vi "Run_Sequence.vi"(0 "Input Sequence":cluster{string, string[], dbl[], dbl}[](array[cluster]), 1 "Alias Table":string[][](array[string]), 2 "API Function Array":cluster{string, "VI Reference":refnum<vi>}[](array[cluster]), 3 "Debug":bool=TRUE, 4 "Resume":bool) -> ()   [LabVIEW 2011]
doc: "This is the highest level VI designed for running growth sequences. It will display all currently running commands, allowing the user to switch between them to view their various statuses. Additionally, if the current command calls for user input before continuing, this VI will display a \"Continue?\" button and enable the \"Waiting for Input...\" indicator. \"Abort Sequence\" will terminate the sequence regardless of the current position and reinitialize the MOCVD system, while \"Pause Sequence\" will end the sequence while leaving the current external hardware state intact. This allows the user to return to the editor, make any applicable changes, and resume the sequence where it was left off."
uses:
  <vilib>/Platform/TimedLoop/XDataNode/nitl_modes.ctl
  <vilib>/Platform/TimedLoop/XDataNode/timing_clust.ctl
  <vilib>/Platform/TimedLoop/XDataNode/wakeup.ctl
  low_level_proc/globals.vi
  Flow_Globals.vi
  <vilib>/Platform/TimedLoop/XDataNode/XDataNode.xnode
  <vilib>/Platform/TimedLoop/XDataNode/XDNodeRunTimeDep.lvlib
panel:
  out "Prev":string
  out "Ended Loop":cluster{string, "Position":i32}[](array[cluster])
  in  "Log/Flow Tabs":T1(tab)=enum."Flow Targets"
  out "Log":string
  out "As":dbl caption="As (0-10 sscm)"
  out "P":dbl caption="P (0-100 sscm)"
  out "In":dbl caption="In (0-10 sscm)"
  out "Ga 3":dbl caption="Ga 3 (0-1000 sscm)"
  out "Ga 2":dbl caption="Ga 2 (0-10 sscm)"
  out "Ga 1":dbl caption="Ga 1 (0-10 sscm)"
  out "Al":dbl caption="Al (0-100 sscm)"
  out "N2":dbl caption="N2 (0-10 slm)"
  out "H2":dbl caption="H2 (0-10 slm)"
  in  "H2/N2 View":bool
  out "As A":dbl caption="As (0-10 sscm)"
  out "P A":dbl caption="P (0-100 sscm)"
  out "In A":dbl caption="In (0-10 sscm)"
  out "Ga 3 A":dbl caption="Ga 3 (0-1000 sscm)"
  out "Ga 2 A":dbl caption="Ga 2 (0-10 sscm)"
  out "Ga 1 A":dbl caption="Ga 1 (0-10 sscm)"
  out "Al A":dbl caption="Al (0-100 sscm)"
  out "N2 A":dbl caption="N2 (0-10000 sscm)"
  out "H2 A":dbl caption="H2 (0-10000 sscm)"
  in  "Heater":bool
  in  "Spinner":bool
  in  "HS Remote":bool caption="Remote"
  out "Position":i32
  out "Ping Time":dbl
  out "Waiting for Input...":bool
  in  "Display Tabs":enum32{"Default", "Time", "Temperature", "Loop"}(tab)
  out "Total Time":u8(slide) caption="Total Time:" scale=0.0..100.0
  out "CE Time":u8(slide) caption="Event Time:" scale=0.0..100.0
  out "Total Time Remaining String":string="00:00" caption="Remaining:"
  out "CE Time Remaining String":string="00:00" caption="Remaining:"
  out "Current Event:":string
  out "Current Temperature (C)":dbl
  out "Target (C)":dbl
  out "Temperature":u8(slide) caption="Temperature:" scale=0.0..100.0
  out "Iteration":string
  in  "Status Tabs":enum32{"Default", "Status", "Prompt"}(tab)
  out "Comment:":string
  out "Selected Event:":string
  in  "Go To Next Step":bool
  out "Prompt:":string
  in  "Continue":bool
  in  "Active Events":i32(listbox)=-1
  in  "Abort":bool
  in  "Pause":bool
  out "Error Out":errorcluster caption="error out"
  out "Running":bool caption="Sequence in Progress..."
  # "Loop Iteration:"
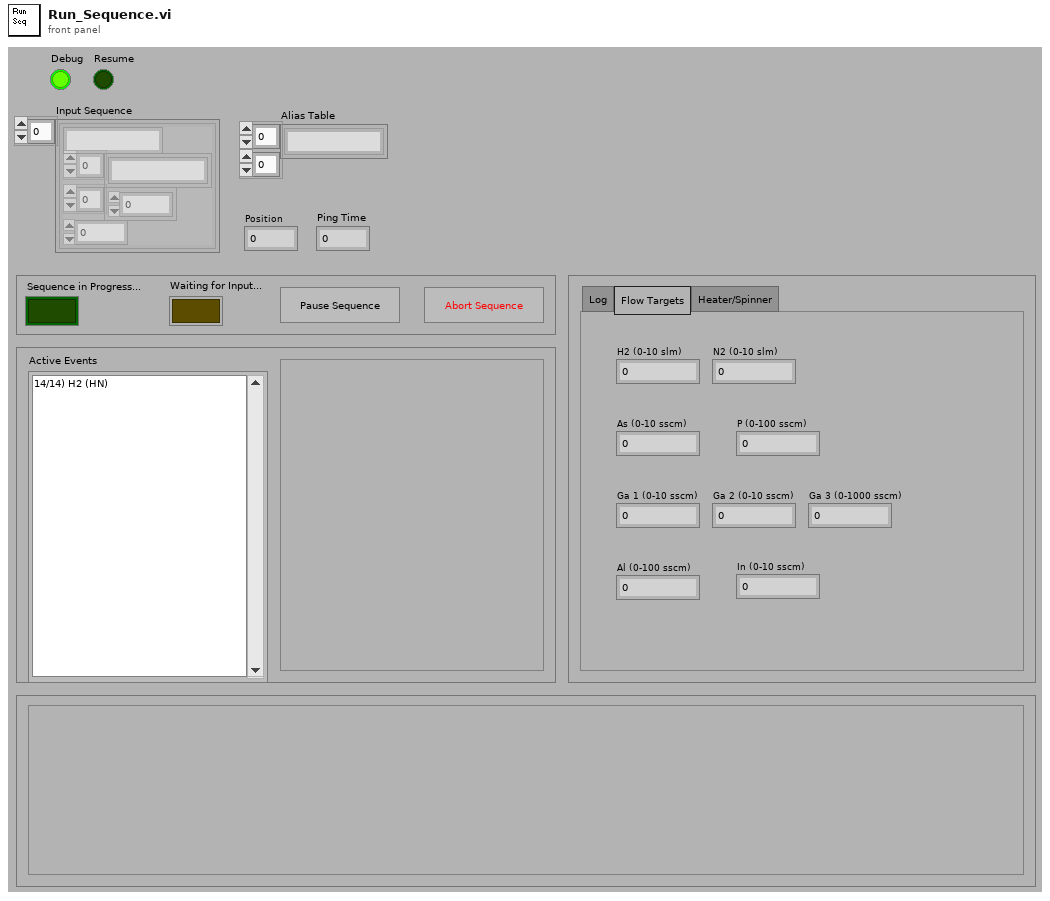
[diagram p1: front panel]
types:
  T1 = enum32{"Log", "Flow Targets", "Detected Flows", "Heater/Spinner"}
  T2 = typedef "XDNodeRunTimeDep.lvlib/nitl_modes.ctl" = enum32{"No Change", "Process missed periods, maintain original phase", "Discard missed periods, maintain original phase", "Process missed periods, ignore original phase", "Discard missed periods, ignore original phase"}
  T3 = enum8{"Enabled", "Disabled", "Disabled and Grayed Out"}
  T4 = typedef "XDNodeRunTimeDep.lvlib/timing_clust.ctl" = cluster{"Expected End [f-1]":u64, "Actual End [f-1]":u64, "Finished Late? [f-1]":bool, "Expected End [i-1]":u64, "Actual End [i-1]":u64, "Finished Late? [i-1]":bool, "Expected Start [i]":u64, "Actual Start [i]":u64, "Expected Start [f]":u64, "Actual Start [f]":u64, "Source Name":string, "Structure Name":string, "Period":i64, "Deadline":i64, "Offset":i64, "Start":i64, "Priority":i32, "Timeout":i32, "Mode":T2, "Wakeup Reason":T5, "Error":errorcluster, "Source Type":string, "Secondary Source Type":string, "Global End Time":u64, "Global Start Time":u64, "Frame Duration":u64, "Iteration Duration":u64, "Assigned CPU":i32, "I/O Scan Engine Mode":u32}
  T5 = typedef "XDNodeRunTimeDep.lvlib/wakeup.ctl" = enum32{"Normal", "Aborted", "Asynchronous wakeup", "Timing source error", "Timed loop error", "Timeout"}
  T6 = enum16{"Normal", "Blocking", "Wait for Input", "Loop"}
  T7 = cluster{"Argument List Out":string[], "Status Out":string}[]
  T8 = cluster{"Total Time Remaining":dbl, "Total Time":dbl, "Current Time Remaining":dbl, "Current Event Time":dbl}
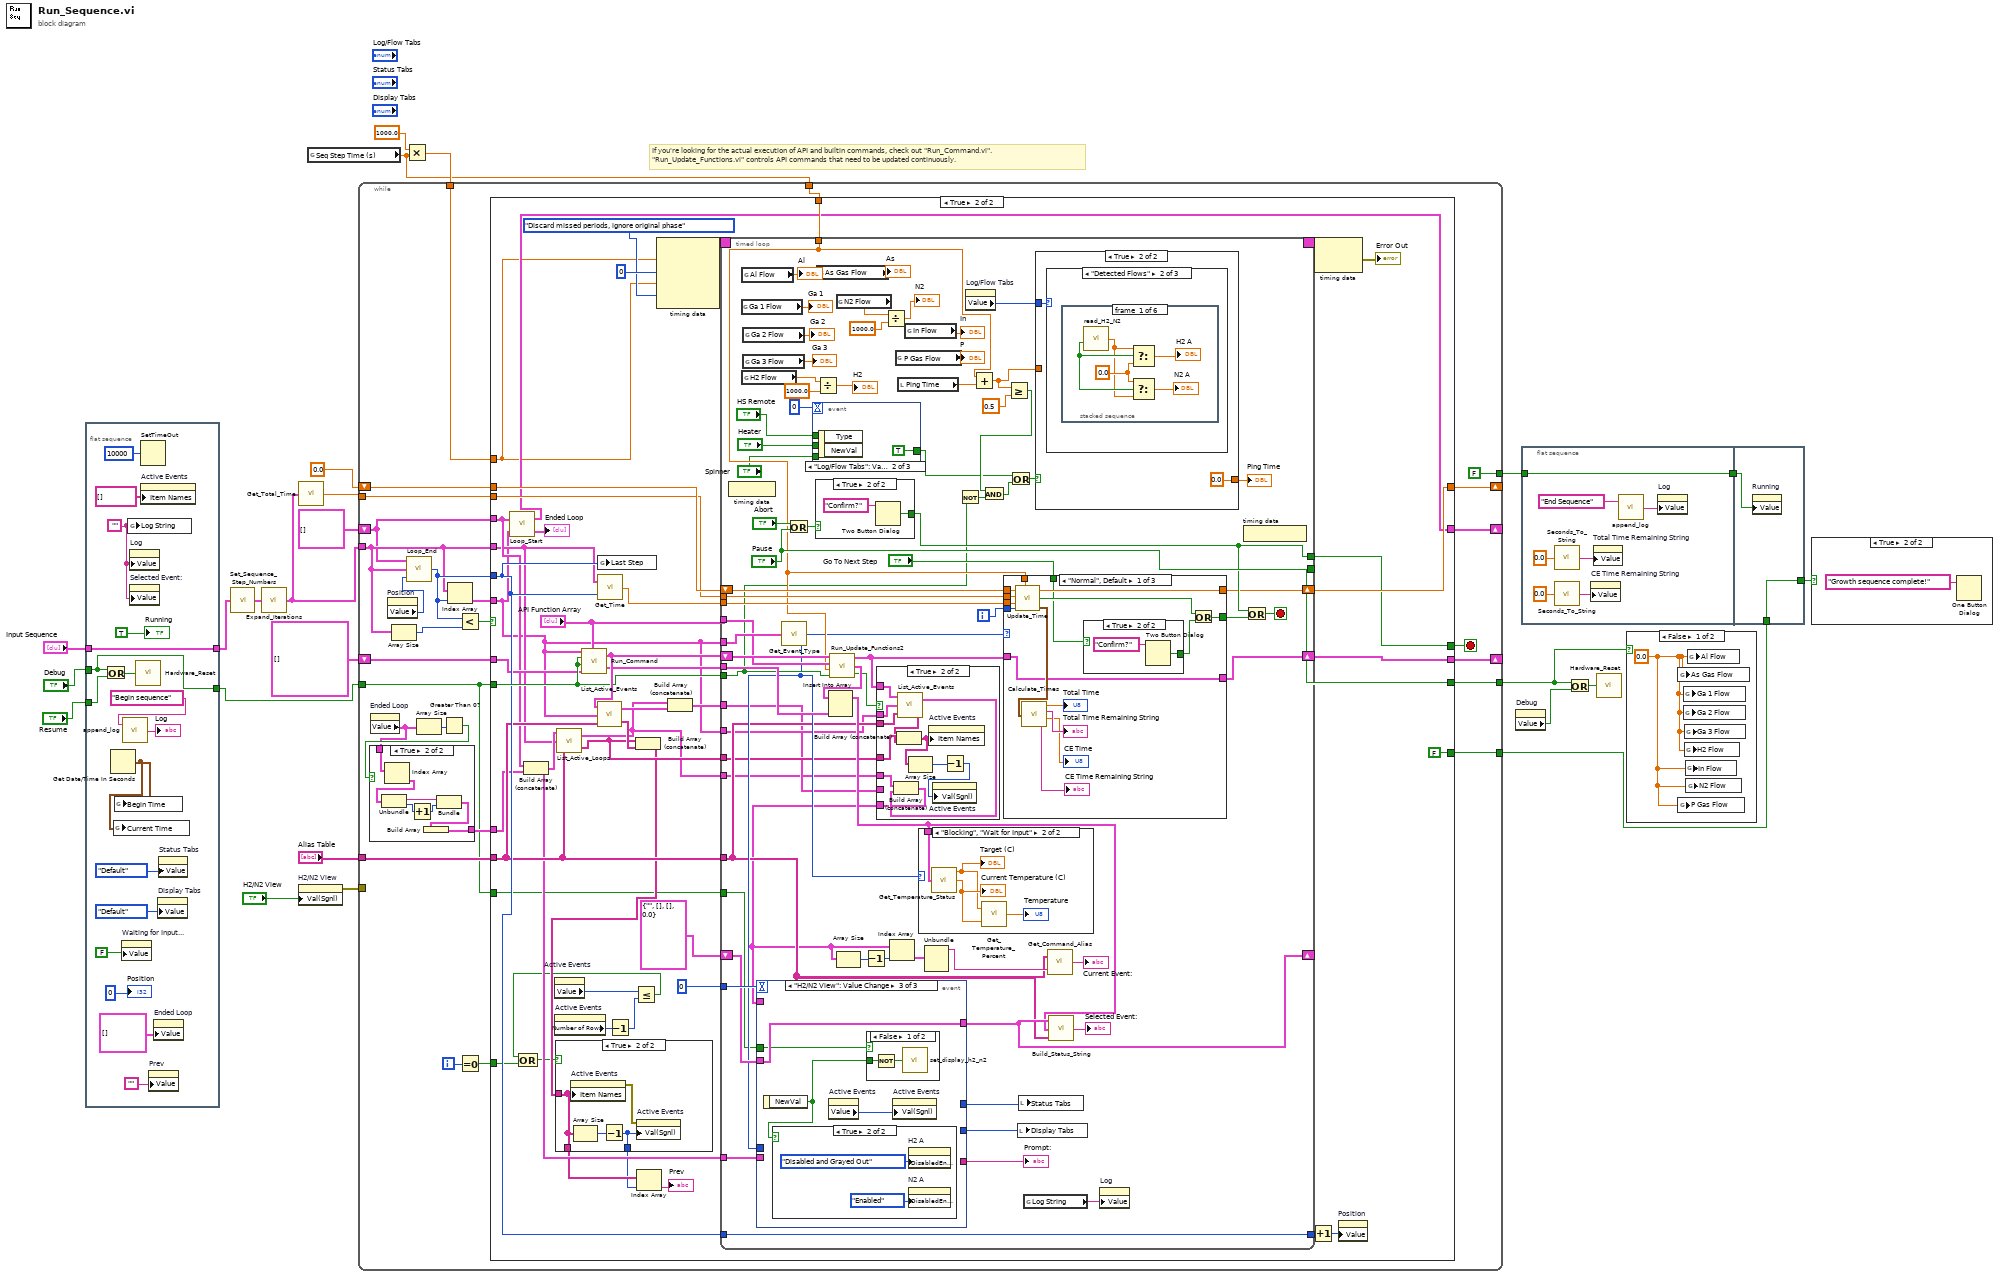
[diagram p0: block diagram]
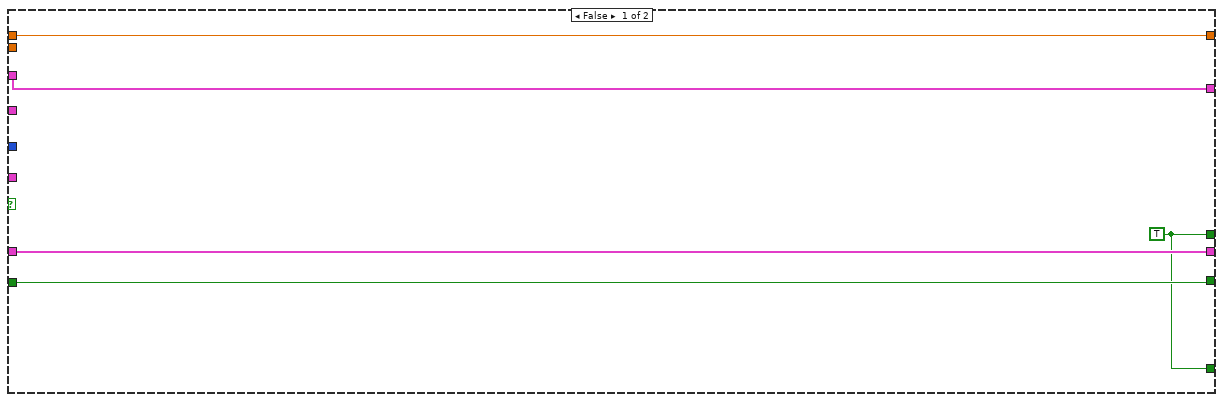
[diagram p4: hidden frame]
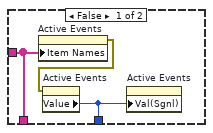
[diagram p5: hidden frame]
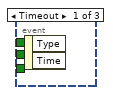
[diagram p7: hidden frame]
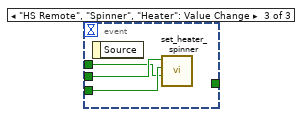
[diagram p8: hidden frame]
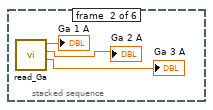
[diagram p12: hidden frame]
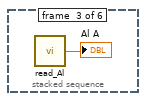
[diagram p13: hidden frame]
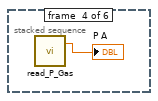
[diagram p14: hidden frame]
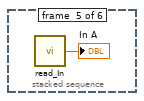
[diagram p15: hidden frame]
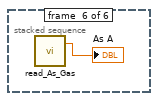
[diagram p16: hidden frame]
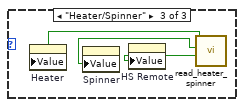
[diagram p17: hidden frame]
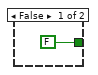
[diagram p18: hidden frame]
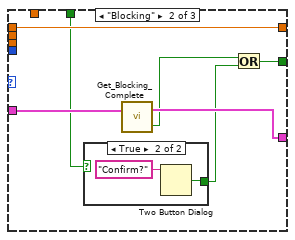
[diagram p19: hidden frame]
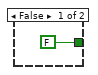
[diagram p20: hidden frame]
diagram:
  # "If you're looking for the actual execution of API and builtin commands, check out \"Run_Command.vi\".\n\"Run_Update_Functions.vi\" controls API commands that need to be updated continuously."
  n1 = flat-sequence {
    tunnel: [w41] -> w3
    tunnel: "Input Sequence" -> [w41]
    tunnel: "Debug" -> [w29]
    tunnel: [w29] -> w19
    tunnel: "Resume" -> [w31]
    frame #0 {
      w36 = ""
      n2 = Or(x=w29, y=w31) -> (x .or. y?=w30:bool)
      n3 = Get Date/Time In Seconds() -> (seconds since 1Jan1904=w37:timestamp)
      n4 = global write "globals.vi" "Current Time"(w37) -> ()
      n5 = global write "globals.vi" "Begin Time"(w37) -> ()
      n6 = property on="Waiting for Input..." class="Bool (strict)"("Value"=FALSE ("Waiting for Input...")) -> ()  [unwired: 2 in, 2 out]
      n7 = call "append_log.vi"("New Log String"="Begin sequence") -> ("Log"=→"Log":string)  [unwired: 1 in]
      n8 = global write "globals.vi" "Log String"(w36) -> ()
      n9 = property on="Log" class="Str"("Value"=w36) -> ()  [unwired: 2 in, 2 out]
      n10 = property on="Selected Event:" class="Str"("Value"=w36) -> ()  [unwired: 2 in, 2 out]
      n11 = call "Hardware_Reset.vi"("Debug"=w30) -> ()  [unwired: 1 out]
      n12 = SetTimeOut(1:10000 ("new timeout (10000)")) -> ()  [unwired: 1 out]
      n13 = property on="Active Events" class="LstBox (strict)"("Item Names"=string[] []) -> ()  [unwired: 2 in, 2 out]
      n14 = property on="Prev" class="Str"("Value"="") -> ()  [unwired: 2 in, 2 out]
      n15 = property on="Ended Loop" class="Arr (strict)"("Value"=cluster{string, "Position":i32}[] [] ("Ended Loop")) -> ()  [unwired: 2 in, 2 out]
      n16 = property on="Display Tabs" class="TabCtl (strict)"("Value"=enum32{"Default", "Time", "Temperature"}."Default" ("Display Tabs")) -> ()  [unwired: 2 in, 2 out]
      n17 = property on="Status Tabs" class="TabCtl (strict)"("Value"=enum32{"Default", "Status", "Prompt"}."Default" ("Status Tabs")) -> ()  [unwired: 2 in, 2 out]
      "Running" <- TRUE ("Sequence in Progress...")
      "Position" <- 0 ("Position")
    }
  }
  n18 = call "Set_Sequence_Step_Numbers.vi"("Input Sequence"=w3) -> ("Output Sequence"=w4:cluster{string, string[], dbl[], dbl}[])
  n19 = call "Expand_Iterations.vi"("Input Sequence"=w4) -> ("Output Sequence"=w9:cluster{string, string[], dbl[], dbl}[])
  n20 = property on="H2/N2 View" class="Bool (strict)"("Val(Sgnl)"="H2/N2 View") -> (error out=w2:errorcluster)  [unwired: 2 in, 1 out]
  n21 = call "Get_Total_Time.vi"("Input Sequence"=w9) -> ("Total Time"=w24:dbl)
  n22 = global read "globals.vi" "Seq Step Time (s)"() -> (w12:dbl)
  n23 = Multiply(x=1000.0, y=w12) -> (x*y=w14:dbl)
  n24 = while {
    tunnel: w24 -> [w66]
    tunnel: [FALSE ("Sequence in Progress...")] -> w20
    tunnel: w9 -> [w53]
    shift-right: [w67] -> _
    shift-left: 0.0 -> [w68]
    tunnel: [w65] -> w5
    shift-right: [w64] -> _
    shift-left: cluster{string, string[], dbl[], dbl}[] [] ("Update Functions Out") -> [w62]
    tunnel: w19 -> [w42]
    tunnel: w14 -> [w63]
    tunnel: "Alias Table" -> [w61]
    tunnel: w12 -> [w60]
    shift-right: [w58] -> _
    shift-left: cluster{string, "Position":i32}[] [] ("appended array") -> [w51]
    tunnel: [w50] -> w8
    tunnel: w2 -> [_]
    i -> [w44]
    stop <- w49 stop-if-true
    n25 = property on="Ended Loop" class="Arr (strict)"() -> ("Value"=w46:cluster{string, "Position":i32}[])  [unwired: 2 in, 2 out]
    n26 = property on="Position" class="DigNum (strict)"() -> ("Value"=w59:i32)  [unwired: 2 in, 2 out]
    n27 = Array Size(array=w53) -> (size(s)=w52:i32)
    n28 = call "Loop_End.vi"("Position In"=w59, "Input Sequence"=w53, "Loop Count In"=w51) -> ("Position Out"=w54:i32)
    n29 = Array Size(array=w46) -> (size(s)=w48:i32)
    n30 = Greater Than 0?(x=w48) -> (x > 0?=w47:bool)
    n31 = case shown="True" w47 {
      tunnel: w46 -> [w69 w76]
      tunnel: [w69 w70] -> w45
      frame False {
      }
      frame True {
        n32 = Index Array(array=w76) -> (element=w75:cluster{string, "Position":i32})  [unwired: 1 in]
        n33 = Unbundle(w75) -> (w72:string, "Position"=w74:i32)
        n34 = Increment(x=w74) -> (x+1=w73:i32)
        n35 = Bundle(w72, w73) -> (w71:cluster{string, i32})  [unwired: 1 in]
        n36 = Build Array(w71) -> (w70:cluster{string, i32}[])
      }
    }
    n37 = Index Array(array=w53, index=w54) -> (element=w56:cluster{string, string[], dbl[], dbl})
    n38 = Less?(x=w54, y=w52) -> (x < y?=w55:bool)
    n39 = Equal To 0?(x=w44) -> (x = 0?=w43:bool)
    n40 = case shown="True" w55 {
      tunnel: w68 -> [w78 w128]
      tunnel: [w78 w127] -> w67
      tunnel: w66 -> [_ w126]
      tunnel: [w79 w125] -> w65
      tunnel: [w81 w124] -> w64
      tunnel: w63 -> [_ w106]
      tunnel: w62 -> [w81 w105]
      tunnel: w61 -> [_ w104]
      tunnel: w60 -> [_ w117]
      tunnel: w42 -> [w79 w115]
      tunnel: w53 -> [_ w97]
      tunnel: w54 -> [_ w111]
      tunnel: w51 -> [w80 w103]
      tunnel: [w80 w108] -> w58
      tunnel: [w77 w112] -> w49
      tunnel: w56 -> [_ w92]
      tunnel: [w77 FALSE ("T button?")] -> w50
      tunnel: w45 -> [_ w102]
      tunnel: w43 -> [_ w94]
      tunnel: w42 -> [_ w82]
      frame False {
        w77 = TRUE ("T button?")
      }
      frame True {
        n41 = call "Loop_Start.vi"("Command"=w92, "Loop Count In"=w103) -> ("Ended Loop"=→"Ended Loop":cluster{string, "Position":i32}[], "Loop Count Out"=w108:cluster{string, "Position":i32}[])
        n42 = Build Array (concatenate)(w103, w102) -> (w98:cluster{string, "Position":i32}[])
        n43 = property on="Active Events" class="LstBox (strict)"() -> ("Value"=w85:i32)  [unwired: 2 in, 2 out]
        n44 = property on="Active Events" class="LstBox (strict)"() -> ("Number of Rows"=w95:u32)  [unwired: 2 in, 2 out]
        n45 = call "List_Active_Loops.vi"("Alias Table"=w104, "Input Sequence"=w97, "Loop Count In"=w98) -> ("Item List"=w93:string[], "Loops Out"=w87:cluster{string, string[], dbl[], dbl}[])
        n46 = call "Run_Command.vi"("Event"=w92, "Debug Mode"=w115, "Realtime Debug"=w115, "Update Functions In"=w105, "API Function Array"="API Function Array") -> ("Update Functions Out"=w118:cluster{string, string[], dbl[], dbl}[], "Status Array"=w114:cluster{string[], "Status Out":string}[])
        n47 = call "List_Active_Events.vi"("Alias Table"=w104, "Current Event"=w92, "Update Functions In"=w118) -> ("Item List"=w101:string[], "Update Functions Out"=w100:cluster{string, string[], dbl[], dbl}[])
        n48 = global write "globals.vi" "Last Step"(w111) -> ()
        n49 = call "Get_Time.vi"("Index"=w111, "Input Sequence"=w97) -> ("Time (s)"=w123:dbl)
        n50 = Decrement(x=w95) -> (x-1=w84:u32)
        n51 = Less Or Equal?(x=w85, y=w84) -> (x <= y?=w83:bool)
        n52 = Compound Arithmetic op=OR(w83, w94) -> (w86:bool)
        n53 = Build Array (concatenate)(w93, w101) -> (w91:string[])
        n54 = case shown="True" w86 {
          tunnel: w91 -> [w132 w135]
          tunnel: [w132 w135] -> w89
          tunnel: [w131 w134] -> w88
          frame False {
            n55 = property on="Active Events" class="LstBox (strict)"("Item Names"=w132) -> (error out=w133:errorcluster)  [unwired: 2 in, 1 out]
            n56 = property on="Active Events" class="LstBox (strict)"(error in=w133) -> ("Value"=w131:i32)  [unwired: 1 in, 2 out]
            n57 = property on="Active Events" class="LstBox (strict)"("Val(Sgnl)"=w131) -> ()  [unwired: 2 in, 2 out]
          }
          frame True {
            n58 = property on="Active Events" class="LstBox (strict)"("Item Names"=w135) -> (error out=w136:errorcluster)  [unwired: 2 in, 1 out]
            n59 = Array Size(array=w135) -> (size(s)=w137:i32)
            n60 = Decrement(x=w137) -> (x-1=w134:i32)
            n61 = property on="Active Events" class="LstBox (strict)"(error in=w136, "Val(Sgnl)"=w134) -> ()  [unwired: 1 in, 2 out]
          }
        }
        n62 = Index Array(array=w89, index=w88) -> (element=→"Prev":string)
        n63 = node-c288(w106, i64 0 ("Offset"), w106, nitl_modes."Discard missed periods, ignore original phase" ("Mode")) -> (w130:T4)
        n64 = Build Array (concatenate)(w87, w100) -> (w99:cluster{string, string[], dbl[], dbl}[])
        n65 = timed-loop {
          timing: w130 -> [_]
          timing-out: [_] -> w129
          tunnel: w123 -> [w197]
          tunnel: w126 -> [w198]
          shift-right: [w196] -> w127
          shift-left: w128 -> [w199]
          tunnel: [w207] -> w112
          tunnel: ["Pause"] -> w125
          shift-right: [w191] -> w124
          shift-left: w118 -> [w192]
          tunnel: w115 -> [w178]
          tunnel: 0 -> [w206]
          tunnel: w104 -> [w153]
          shift-right: [w185] -> _
          shift-left: cluster{string, string[], dbl[], dbl} {"", [], [], 0.0} -> [w202]
          tunnel: w92 -> [w201]
          tunnel: w99 -> [w150]
          tunnel: "API Function Array" -> [w190]
          tunnel: w117 -> [w180]
          tunnel: w114 -> [w183]
          tunnel: w111 -> [w174]
          tunnel: [w174] -> w113
          tunnel: w98 -> [w156]
          tunnel: w93 -> [w152]
          tunnel: w92 -> [w151]
          tunnel: w87 -> [w148]
          tunnel: w82 -> [w141]
          i -> [w181]
          stop <- w208 stop-if-true
          n66 = node-c288() -> ()  [unwired: 1 out]
          n67 = global read "Flow_Globals.vi" "Ga 1 Flow"() -> (→"Ga 1":dbl)
          n68 = global read "Flow_Globals.vi" "Al Flow"() -> (→"Al":dbl)
          n69 = global read "Flow_Globals.vi" "H2 Flow"() -> (w147:dbl)
          n70 = global read "Flow_Globals.vi" "Ga 2 Flow"() -> (→"Ga 2":dbl)
          n71 = global read "Flow_Globals.vi" "Ga 3 Flow"() -> (→"Ga 3":dbl)
          n72 = call "Get_Event_Type.vi"("Event"=w201) -> ("Event Type"=w177:T6)
          n73 = Or(x="Abort", y="Pause") -> (x .or. y?=w189:bool)
          n74 = event shown="[1] \"Log/Flow Tabs\": Value Change" {
            selector: _ -> [_ _ _]
            dyn-events: _ -> [_ _ _]
            timeout: 0 -> [_ _ _]
            tunnel: [_ TRUE _] -> w161
            tunnel: "HS Remote" -> [_ _ w224]
            tunnel: "Spinner" -> [_ _ w226]
            tunnel: "Heater" -> [_ _ w225]
            event Timeout {
              n75 = event-data() -> ()  [unwired: 1 in, 2 out]
            }
            event "Log/Flow Tabs": Value Change {
              n76 = event-data() -> ()  [unwired: 1 in, 2 out]
            }
            event "HS Remote", "Spinner", "Heater": Value Change {
              n77 = event-data() -> ()  [unwired: 1 in, 1 out]
              n78 = call "set_heater_spinner.vi"("Remote"=w224, "Spinner"=w226, "Heater"=w225) -> ()  [unwired: 7 out]
            }
          }
          n79 = Divide(x=w147, y=1000.0) -> (x/y=→"H2":dbl)
          n80 = case shown="True" w189 {
            tunnel: [FALSE ("T button?") w334] -> w207
            frame False {
            }
            frame True {
              n81 = Two Button Dialog(message="Confirm?") -> (T button?=w334:bool)  [unwired: 2 out]
            }
          }
          n82 = global read "Flow_Globals.vi" "As Gas Flow"() -> (→"As":dbl)
          n83 = call "Run_Update_Functions2.vi"("Debug Mode"=w178, "Time Delta (s)"=w180, "API Function Array"=w190, "Update Functions In"=w192) -> ("Refresh"=w155:bool, "Status Array"=w184:T7, "Update Functions Out"=w154:cluster{string, string[], dbl[], dbl}[])
          n84 = Insert Into Array(array=w184, new element=w183) -> (w176:T7)  [unwired: 1 in]
          n85 = global read "Flow_Globals.vi" "N2 Flow"() -> (w142:dbl)
          n86 = case shown="True" w155 {
            tunnel: w154 -> [_ w215]
            tunnel: w153 -> [_ w221]
            tunnel: w152 -> [_ w222]
            tunnel: w151 -> [_ w220]
            tunnel: w150 -> [w211 _]
            tunnel: [w211 w212] -> w149
            tunnel: w148 -> [_ w214]
            frame False {
            }
            frame True {
              n87 = call "List_Active_Events.vi"("Alias Table"=w221, "Current Event"=w220, "Update Functions In"=w215) -> ("Item List"=w219:string[], "Update Functions Out"=w213:cluster{string, string[], dbl[], dbl}[])
              n88 = Build Array (concatenate)(w214, w213) -> (w212:cluster{string, string[], dbl[], dbl}[])
              n89 = Build Array (concatenate)(w222, w219) -> (w216:string[])
              n90 = Array Size(array=w216) -> (size(s)=w218:i32)
              n91 = property on="Active Events" class="LstBox (strict)"("Item Names"=w216) -> ()  [unwired: 2 in, 2 out]
              n92 = Decrement(x=w218) -> (x-1=w217:i32)
              n93 = property on="Active Events" class="LstBox (strict)"("Val(Sgnl)"=w217) -> ()  [unwired: 2 in, 2 out]
            }
          }
          n94 = event shown="[2] \"H2/N2 View\": Value Change" {
            selector: _ -> [_ _ _]
            dyn-events: _ -> [_ _ _]
            timeout: w206 -> [_ _ _]
            tunnel: w149 -> [_ w298 _]
            tunnel: [w287 w291 w326] -> w185
            tunnel: w202 -> [w287 _ w326]
            tunnel: [w284 w296 _] -> w193
            tunnel: [w286 w295 _] -> w187
            tunnel: [w285 w294 _] -> w188
            tunnel: w177 -> [_ w293 _]
            tunnel: w156 -> [_ w288 _]
            tunnel: w141 -> [_ _ w323]
            event Timeout {
              n95 = event-data() -> ()  [unwired: 3 out]
              n96 = property on="Status Tabs" class="TabCtl (strict)"() -> ("Value"=w286:enum32{"Default", "Status", "Prompt"})  [unwired: 2 in, 2 out]
              n97 = property on="Display Tabs" class="TabCtl (strict)"() -> ("Value"=w285:enum32{"Default", "Time", "Temperature", "Loop"})  [unwired: 2 in, 2 out]
              n98 = property on="Prompt:" class="Str"() -> ("Value"=w284:string)  [unwired: 2 in, 2 out]
            }
            event "Active Events": Value Change {
              n99 = event-data() -> ()  [unwired: 2 out]
              n100 = Index Array(array=w298, index="Active Events") -> (element=w291:cluster{string, string[], dbl[], dbl})
              n101 = Unbundle(w291) -> (w290:string[])  [unwired: 3 out]
              n102 = call "Get_Text_Argument.vi"("Argument"="Comment", "Argument List"=w290) -> ("Text"=→"Comment:":string)
              n103 = call "Get_Event_Type.vi"("Event"=w291) -> ("Event Type"=w297:T6)
              n104 = case shown="\"Loop\"" w297 {
                tunnel: w291 -> [w305 w314 w320]
                tunnel: [_ w313 _] -> w296
                tunnel: [w301 w312 enum32{"Default", "Status", "Prompt"}."Default" ("Status Tabs")] -> w295
                tunnel: [w300 enum32{"Default", "Time", "Temperature", "Loop"}."Temperature" ("Display Tabs") enum32{"Default", "Time", "Temperature", "Loop"}."Loop" ("Display Tabs")] -> w294
                tunnel: w293 -> [_ w311 _]
                tunnel: w288 -> [_ _ w319]
                frame "Normal", Default {
                  n105 = Unbundle(w305) -> (w304:string)  [unwired: 3 out]
                  n106 = String Length(string=w304) -> (length=w303:i32)
                  n107 = Greater Than 0?(x=w303) -> (x > 0?=w302:bool)
                  n108 = case shown="True" w302 {
                    tunnel: [enum32{"Default", "Status", "Prompt"}."Status" ("Status Tabs") enum32{"Default", "Status", "Prompt"}."Status" ("Status Tabs")] -> w301
                    tunnel: [enum32{"Default", "Time", "Temperature", "Loop"}."Time" ("Display Tabs") enum32{"Default", "Time", "Temperature", "Loop"}."Time" ("Display Tabs")] -> w300
                    frame False {
                    }
                    frame True {
                    }
                  }
                }
                frame "Blocking", "Wait for Input" {
                  n109 = call "Get_Prompt.vi"("Event"=w314) -> ("Prompt"=w313:string)
                  n110 = case shown="\"Blocking\"" w311 {
                    tunnel: [enum32{"Default", "Status", "Prompt"}."Default" ("Status Tabs") enum32{"Default", "Status", "Prompt"}."Status" ("Status Tabs") enum32{"Default", "Status", "Prompt"}."Prompt" ("Status Tabs")] -> w312
                    frame "Normal", Default {
                    }
                    frame "Blocking" {
                    }
                    frame "Wait for Input" {
                    }
                  }
                }
                frame "Loop" {
                  n111 = call "Get_Loop_Iteration.vi"("Loop Count"=w319, "Loop Event"=w320) -> ("Iteration Descriptor"=→"Iteration":string)
                }
              }
            }
            event "H2/N2 View": Value Change {
              n112 = event-data() -> ("NewVal"=w324:bool)  [unwired: 1 out]
              n113 = case shown="True" w324 {
                frame False {
                  n114 = property on="H2 A" class="DigNum (strict)"("DisabledEnum"=T3."Enabled" ("Disabled")) -> ()  [unwired: 2 in, 2 out]
                  n115 = property on="N2 A" class="DigNum (strict)"("DisabledEnum"=T3."Disabled and Grayed Out" ("Disabled")) -> ()  [unwired: 2 in, 2 out]
                }
                frame True {
                  n116 = property on="H2 A" class="DigNum (strict)"("DisabledEnum"=T3."Disabled and Grayed Out" ("Disabled")) -> ()  [unwired: 2 in, 2 out]
                  n117 = property on="N2 A" class="DigNum (strict)"("DisabledEnum"=T3."Enabled" ("Disabled")) -> ()  [unwired: 2 in, 2 out]
                }
              }
              n118 = property on="Active Events" class="LstBox (strict)"() -> ("Value"=w325:i32)  [unwired: 2 in, 2 out]
              n119 = case shown="False" w323 {
                tunnel: w324 -> [w328 _]
                frame False {
                  n120 = Not(x=w328) -> (.not. x?=w327:bool)
                  n121 = call "set_display_h2_n2.vi"("Display H2 or N2"=w327) -> ()
                }
                frame True {
                }
              }
              n122 = property on="Active Events" class="LstBox (strict)"("Val(Sgnl)"=w325) -> ()  [unwired: 2 in, 2 out]
            }
          }
          "Prompt:" <- w193
          n123 = Array Size(array=w149) -> (size(s)=w203:i32)
          n124 = Decrement(x=w203) -> (x-1=w204:i32)
          n125 = Divide(x=w142, y=1000.0) -> (x/y=→"N2":dbl)
          n126 = Index Array(array=w149, index=w204) -> (element=w205:cluster{string, string[], dbl[], dbl})
          n127 = global read "Flow_Globals.vi" "P Gas Flow"() -> (→"P":dbl)
          n128 = local read "Ping Time"() -> (w139:dbl)
          n129 = global read "Flow_Globals.vi" "In Flow"() -> (→"In":dbl)
          n130 = case shown="\"Blocking\", \"Wait for Input\"" w177 {
            tunnel: w176 -> [_ w227]
            frame "Normal", Default {
            }
            frame "Blocking", "Wait for Input" {
              n131 = call "Get_Temperature_Status.vi"("Status Array"=w227) -> ("Setpoint"=w229:dbl, "Temperature"=w230:dbl)  [unwired: 1 out]
              "Target (C)" <- w229
              "Current Temperature (C)" <- w230
              n132 = call "Get_Temperature_Percent.vi"("Temperature"=w230, "Setpoint"=w229) -> ("Temperature Percent"=→"Temperature":dbl)
            }
          }
          n133 = Unbundle(w205) -> (w195:string)  [unwired: 3 out]
          n134 = Not(x=w178) -> (.not. x?=w173:bool)
          n135 = property on="Log/Flow Tabs" class="TabCtl (strict)"() -> ("Value"=w171:T1)  [unwired: 2 in, 2 out]
          n136 = Add(x=w180, y=w139) -> (x+y=w138:dbl)
          n137 = case shown="\"Normal\", Default" w177 {
            tunnel: [w251 w268 w278] -> w200
            tunnel: w199 -> [w260 w274 w283]
            tunnel: w198 -> [w259 _ _]
            tunnel: w197 -> [w258 _ _]
            tunnel: w181 -> [w257 _ _]
            tunnel: [w253 w274 w283] -> w196
            tunnel: w154 -> [w255 w273 w282]
            tunnel: [w255 w272 w282] -> w191
            tunnel: w180 -> [w254 _ _]
            tunnel: "Go To Next Step" -> [w249 w270 w279]
            frame "Normal", Default {
              n138 = call "Update_Time.vi"("Total Time Elapsed In"=w260, "Total Time"=w259, "Current Event Time"=w258, "Iteration"=w257, "Delta Time (s)"=w254) -> ("Total Time Elapsed Out"=w253:dbl, "End"=w252:bool, "Output Times"=w256:T8)
              n139 = call "Calculate_Times.vi"("Input Times"=w256) -> ("Total Percent"=→"Total Time":dbl, "Total String"=→"Total Time Remaining String":string, "Current Percent"=→"CE Time":dbl, "Current String"=→"CE Time Remaining String":string)
              n140 = case shown="True" w249 {
                tunnel: [FALSE ("T button?") w266] -> w250
                frame False {
                }
                frame True {
                  n141 = Two Button Dialog(message="Confirm?") -> (T button?=w266:bool)  [unwired: 2 out]
                }
              }
              n142 = Or(x=w252, y=w250) -> (x .or. y?=w251:bool)
            }
            frame "Blocking" {
              n143 = case shown="True" w270 {
                tunnel: [FALSE ("T button?") w276] -> w271
                frame False {
                }
                frame True {
                  n144 = Two Button Dialog(message="Confirm?") -> (T button?=w276:bool)  [unwired: 2 out]
                }
              }
              n145 = call "Get_Blocking_Complete.vi"("Update Functions In"=w273) -> ("Update Functions Out"=w272:cluster{string, string[], dbl[], dbl}[], "Event Completed"=w269:bool)
              n146 = Or(x=w269, y=w271) -> (x .or. y?=w268:bool)
            }
            frame "Wait for Input" {
              n147 = Not(x="Continue") -> (.not. x?=→"Waiting for Input...":bool)
              n148 = Or(x=w279, y="Continue") -> (x .or. y?=w278:bool)
            }
          }
          n149 = Greater Or Equal?(x=w138, y=0.5) -> (x >= y?=w172:bool)
          n150 = And(x=w172, y=w173) -> (x .and. y?=w163:bool)
          n151 = Or(x=w161, y=w163) -> (x .or. y?=w160:bool)
          n152 = local write "Display Tabs"(w188) -> ()
          n153 = local write "Status Tabs"(w187) -> ()
          n154 = global read "globals.vi" "Log String"() -> (w175:string)
          n155 = case shown="True" w160 {
            tunnel: w171 -> [_ w233]
            tunnel: [w231 0.0 ("H2 Ping Time")] -> w140
            tunnel: w138 -> [w231 _]
            frame False {
            }
            frame True {
              n156 = case shown="\"Detected Flows\"" w233 {
                frame Default {
                }
                frame "Detected Flows" {
                  n157 = stacked-sequence {
                    frame #0 {
                      w236 = 0.0 ("f")
                      n158 = call "read_H2_N2.vi"() -> ("H2N2 Flow Rate"=w234:dbl, "Display H2N2"=w235:bool)  [unwired: 3 out]
                      n159 = Select(t=w234, s=w235, f=w236) -> (s? t:f=→"H2 A":dbl)
                      n160 = Select(t=w236, s=w235, f=w234) -> (s? t:f=→"N2 A":dbl)
                    }
                    frame #1 {
                      n161 = call "read_Ga.vi"() -> ("GAMFC3"=→"Ga 3 A":dbl, "GAMFC2"=→"Ga 2 A":dbl, "GAMFC1"=→"Ga 1 A":dbl)  [unwired: 5 out]
                    }
                    frame #2 {
                      n162 = call "read_Al.vi"() -> ("ALMFC1"=→"Al A":dbl)  [unwired: 4 out]
                    }
                    frame #3 {
                      n163 = call "read_P_Gas.vi"() -> ("P Gas Actual Flow Rate"=→"P A":dbl)  [unwired: 5 out]
                    }
                    frame #4 {
                      n164 = call "read_In.vi"() -> ("INMFC1"=→"In A":dbl)  [unwired: 4 out]
                    }
                    frame #5 {
                      n165 = call "read_As_Gas.vi"() -> ("As Gas Actual Flow Rate"=→"As A":dbl)  [unwired: 5 out]
                    }
                  }
                }
                frame "Heater/Spinner" {
                  n166 = call "read_heater_spinner.vi"() -> ("Heater/Spinner Remote"=w248:bool, "Spinner"=w246:bool, "Heater"=w247:bool)  [unwired: 7 out]
                  n167 = property on="Heater" class="Bool (strict)"("Value"=w247) -> ()  [unwired: 2 in, 2 out]
                  n168 = property on="Spinner" class="Bool (strict)"("Value"=w246) -> ()  [unwired: 2 in, 2 out]
                  n169 = property on="HS Remote" class="Bool (strict)"("Value"=w248) -> ()  [unwired: 2 in, 2 out]
                }
              }
            }
          }
          "Ping Time" <- w140
          n170 = call "Get_Command_Alias.vi"("Command"=w195, "Alias Table"=w153) -> ("Alias"=→"Current Event:":string)
          n171 = call "Build_Status_String.vi"("Alias Table"=w153, "Status Array"=w176, "Event"=w185) -> ("Status"=→"Selected Event:":string)
          n172 = property on="Log" class="Str"("Value"=w175) -> ()  [unwired: 2 in, 2 out]
          n173 = node-c288() -> ()  [unwired: 1 out]
          n174 = Or(x=w207, y=w200) -> (x .or. y?=w208:bool)
        }
        n175 = Increment(x=w113) -> (x+1=w110:i32)
        n176 = node-c288(w129) -> (→"Error Out":errorcluster)
        n177 = property on="Position" class="DigNum (strict)"("Value"=w110) -> ()  [unwired: 2 in, 2 out]
      }
    }
  }
  n178 = property on="Debug" class="Bool (strict)"() -> ("Value"=w6:bool)  [unwired: 2 in, 2 out]
  n179 = flat-sequence {
    tunnel: w20 -> [w348]
    tunnel: [w348] -> w18
    tunnel: w18 -> [w354]
    tunnel: w8 -> [w353]
    tunnel: [w353] -> w17
    frame #0 {
      n180 = call "Seconds_To_String.vi"("Seconds"=0.0) -> ("Output String"=w351:string)
      n181 = call "Seconds_To_String.vi"("Seconds"=0.0) -> ("Output String"=w350:string)
      n182 = property on="CE Time Remaining String" class="Str"("Value"=w350) -> ()  [unwired: 2 in, 2 out]
      n183 = property on="Total Time Remaining String" class="Str"("Value"=w351) -> ()  [unwired: 2 in, 2 out]
      n184 = call "append_log.vi"("New Log String"="End Sequence") -> ("Log"=w346:string)  [unwired: 1 in]
      n185 = property on="Log" class="Str"("Value"=w346) -> ()  [unwired: 2 in, 2 out]
    }
    frame #1 {
      n186 = property on="Running" class="Bool (strict)"("Value"=w354) -> ()  [unwired: 2 in, 2 out]
    }
  }
  n187 = Or(x=w5, y=w6) -> (x .or. y?=w7:bool)
  n188 = call "Hardware_Reset.vi"("Debug"=w7) -> ()  [unwired: 1 out]
  n189 = case shown="False" w5 {
    frame False {
      w355 = 0.0 ("Al Flow")
      n190 = global write "Flow_Globals.vi" "As Gas Flow"(w355) -> ()
      n191 = global write "Flow_Globals.vi" "P Gas Flow"(w355) -> ()
      n192 = global write "Flow_Globals.vi" "Ga 1 Flow"(w355) -> ()
      n193 = global write "Flow_Globals.vi" "Ga 2 Flow"(w355) -> ()
      n194 = global write "Flow_Globals.vi" "Ga 3 Flow"(w355) -> ()
      n195 = global write "Flow_Globals.vi" "H2 Flow"(w355) -> ()
      n196 = global write "Flow_Globals.vi" "In Flow"(w355) -> ()
      n197 = global write "Flow_Globals.vi" "N2 Flow"(w355) -> ()
      n198 = global write "Flow_Globals.vi" "Al Flow"(w355) -> ()
    }
    frame True {
    }
  }
  n199 = case shown="True" w17 {
    frame False {
    }
    frame True {
      n200 = One Button Dialog(message="Growth sequence complete!") -> ()  [unwired: 2 out]
    }
  }
